vi "Get Build Specifications.vi"(8 "Error In":errorcluster, 11 "Project Path":path) -> (0 "Error Out":errorcluster, 2 "BuildSpecification Names":string[](array[string]), 3 "Project Path Out":path)   [LabVIEW 2020]
doc: "Write Build Parametes:\nInput: Project Path (Path), Build Spec to Edit (String), Save Project? (Boolean), Error In\nOutput: Project Path Out (Path)\n\nThis VI finds a specific build in a project and writes the parameters found in EXE Build Properties. Optionally saves the project afterwards.\n\nCreated by Douglas Thor on 2011-12-16, based on work by James W."
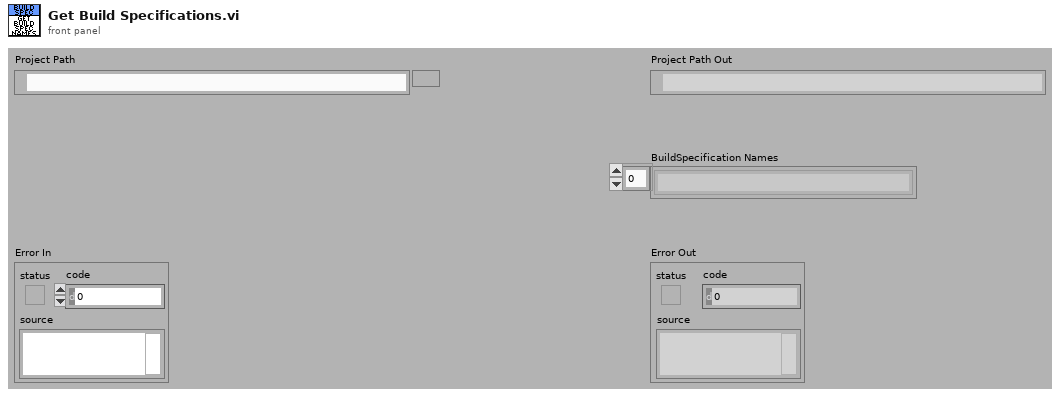
[diagram p1: front panel]
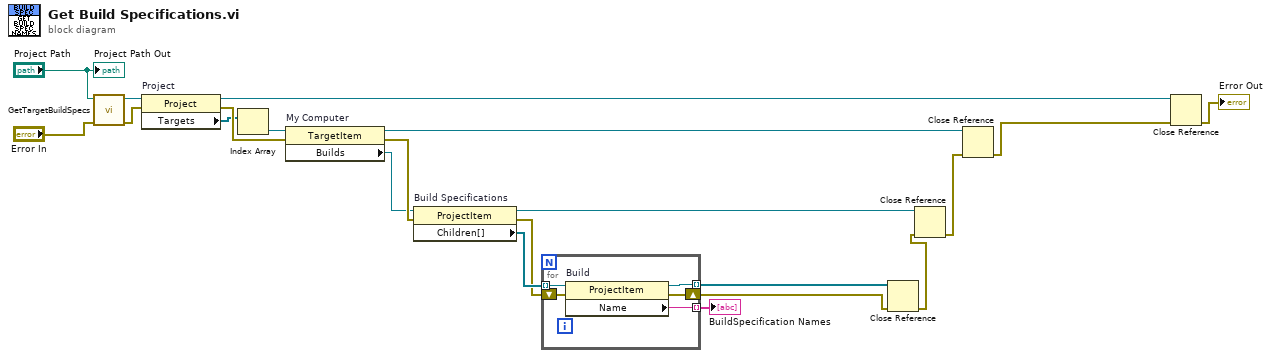
[diagram p0: block diagram]
diagram:
  n1 = call <vilib>:"GetTargetBuildSpecs.vi"("error in (no error)"="Error In", "Path to project"="Project Path") -> ("error out"=w10:errorcluster, "project ref"=w13:refnum<vi>)  [unwired: 7 in, 1 out]
  n2 = property on="Project" class="Project"(reference=w13, error in=w10) -> (reference out=w12:refnum<vi>, error out=w20:errorcluster, "Targets"=w19:refnum<vi>[])
  n3 = Index Array(array=w19) -> (element=w18:refnum<vi>)  [unwired: 1 in]
  n4 = property on="My Computer" class="TargetItem"(reference=w18, error in=w20) -> (reference out=w16:refnum<vi>, error out=w21:errorcluster, "Builds"=w17:refnum<vi>)
  n5 = property on="Build Specifications" class="ProjectItem"(reference=w17, error in=w21) -> (reference out=w5:refnum<vi>, error out=w9:errorcluster, "Children[]"=w14:refnum<vi>[])
  n6 = for {
    tunnel: w14 -> [w26] mode=indexing
    tunnel: [w25] -> w6 mode=indexing
    shift-right: [w23] -> w3
    shift-left: w9 -> [w24]
    tunnel: [w22] -> w4 mode=indexing
    n7 = property on="Build" class="ProjectItem"(reference=w26, error in=w24) -> (reference out=w22:refnum<vi>, error out=w23:errorcluster, "Name"=w25:string)
  }
  "BuildSpecification Names" <- w6
  n8 = Close Reference(reference=w4, error in (no error)=w3) -> (error out=w2:errorcluster)
  n9 = Close Reference(reference=w5, error in (no error)=w2) -> (error out=w15:errorcluster)
  n10 = Close Reference(reference=w16, error in (no error)=w15) -> (error out=w1:errorcluster)
  n11 = Close Reference(reference=w12, error in (no error)=w1) -> (error out=→"Error Out":errorcluster)
  "Project Path Out" <- "Project Path"
